vi "antiRC.vi"(1 "time interval":dbl[](array[numeric]) format="%.2f", 2 "tau":dbl format="%.2f", 3 "in":dbl[](array[numeric]) format="%.2f") -> (0 "out":dbl[](array[numeric]) format="%.2f")   [LabVIEW 2018]
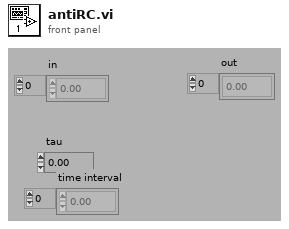
[diagram p1: front panel]
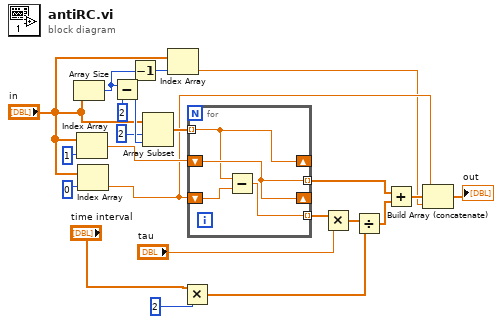
[diagram p0: block diagram]
diagram:
  n1 = Array Size(array="in") -> (size(s)=w6:i32)
  n2 = Index Array(array="in", index=1) -> (element=w8:dbl)
  n3 = Index Array(array="in", index=0) -> (element=w7:dbl)
  n4 = Subtract(x=w6, y=2) -> (x-y=w19:i32)
  n5 = Decrement(x=w6) -> (x-1=w5:i32)
  n6 = Array Subset(array="in", index=2, length=w19) -> (w17:dbl[])
  n7 = Index Array(array="in", index=w5) -> (element=w3:dbl)
  n8 = Multiply(x="time interval", y=2) -> (x*y=w12:dbl[])
  n9 = for {
    shift-right: [w25] -> _
    shift-left: w8 -> [w26]
    shift-right: [w26] -> _
    shift-left: w7 -> [w24]
    tunnel: w17 -> [w25] mode=indexing
    tunnel: [w26] -> w11 mode=indexing
    tunnel: [w23] -> w15 mode=indexing
    n10 = Subtract(x=w25, y=w24) -> (x-y=w23:dbl)
  }
  n11 = Multiply(x=w15, y="tau") -> (x*y=w13:dbl[])
  n12 = Divide(x=w13, y=w12) -> (x/y=w10:dbl[])
  n13 = Add(x=w11, y=w10) -> (x+y=w9:dbl[])
  n14 = Build Array (concatenate)(w7, w9, w3) -> (→"out":dbl[])
